vi "Get Single Reference.vi"(8 "error in (no error)":errorcluster, 10 "Control Name":string, 11 "Controls_Mgr in":refnum<class "Controls_Mgr.lvclass">) -> (0 "error out":errorcluster, 2 "Control Reference":refnum<vi>, 3 "Controls_Mgr out":refnum<class "Controls_Mgr.lvclass">)   [LabVIEW 2015, in "Generic Module Library.lvlib" / "Template G_Module.lvlib" / "Controls_Mgr.lvclass"]
uses:
  Controls_Mgr.lvclass
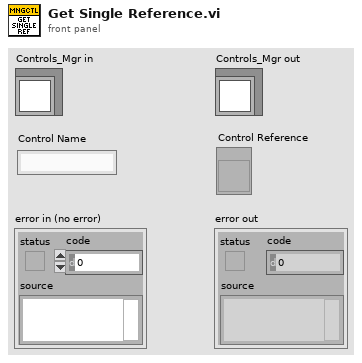
[diagram p1: front panel]
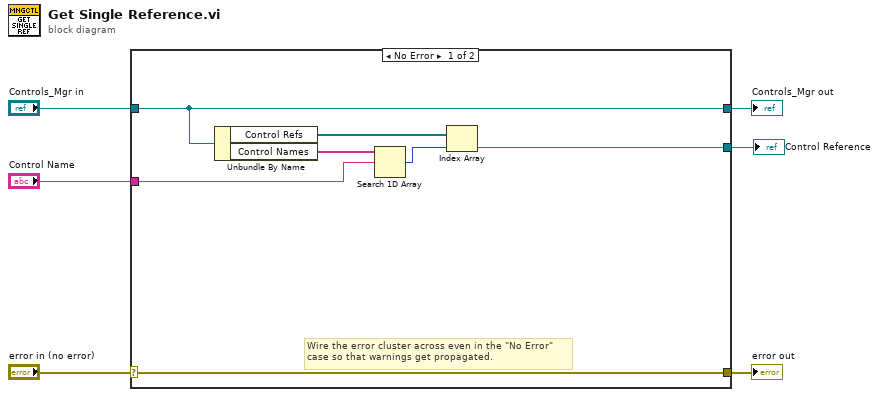
[diagram p0: block diagram]
diagram:
  n1 = case shown="No Error" "error in (no error)" {
    selector: "error in (no error)" -> [w13 w15]
    tunnel: [w13 w15] -> w5
    tunnel: [w12 w14] -> w3
    tunnel: "Controls_Mgr in" -> [w12 w14]
    tunnel: "Control Name" -> [w10 _]
    tunnel: [w7 _] -> w1
    frame No Error {
      # "Wire the error cluster across even in the \"No Error\"\ncase so that warnings get propagated."
      n2 = Unbundle By Name(w12) -> ("Control Refs"=w8:refnum<vi>[], "Control Names"=w11:string[])
      n3 = Search 1D Array(1D array=w11, element=w10) -> (index of element=w9:i32)  [unwired: 1 in]
      n4 = Index Array(array=w8, index=w9) -> (element=w7:refnum<vi>)
    }
    frame Error {
    }
  }
  "error out" <- w5
  "Controls_Mgr out" <- w3
  "Control Reference" <- w1
